vi "TCP-Ping.vi"(0 "IP Address":string, 5 "Port":i32, 11 "error in (no error)":errorcluster) -> (15 "error out":errorcluster)   [LabVIEW 2020]
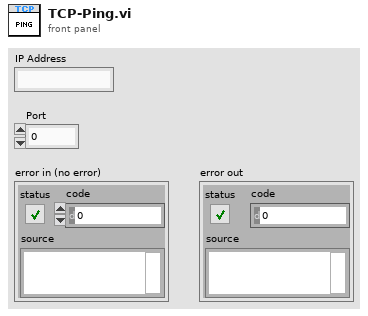
[diagram p1: front panel]
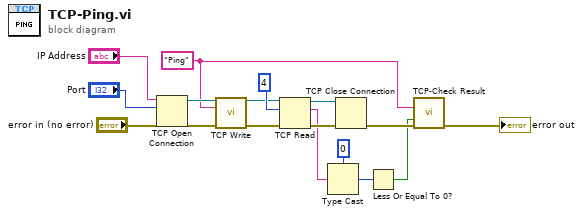
[diagram p0: block diagram]
diagram:
  w6 = "Ping" ("data string")
  n1 = TCP Open Connection(address="IP Address", remote port or service name="Port", error in (no error)="error in (no error)") -> (connection ID=w11:refnum<k5>, error out=w10:errorcluster)  [unwired: 2 in]
  n2 = call "TCP Write.vi"("connection ID"=w11, "data string"=w6, "error in (no error)"=w10) -> ("connection ID out"=w14:refnum<k5>, "error out"=w13:errorcluster)  [unwired: 10 in, 1 out]
  n3 = TCP Read(connection ID=w14, bytes to read=4, error in (no error)=w13) -> (connection ID out=w17:refnum<k5>, data out=w4:string, error out=w16:errorcluster)  [unwired: 2 in]
  n4 = Type Cast(type=0 ("bytes to read"), x=w4) -> (*(type *) &x=w2:i32)
  n5 = TCP Close Connection(connection ID=w17, error in (no error)=w16) -> (error out=w7:errorcluster)  [unwired: 1 in, 1 out]
  n6 = Less Or Equal To 0?(x=w2) -> (x <= 0?=w1:bool)
  n7 = call "TCP-Check Result.vi"("command"=w6, "invalid response"=w1, "error IO"=w7) -> ("error out"=→"error out":errorcluster)  [unwired: 12 in]
